vi "GoDef.vi"(8 "error in (no error)":errorcluster, 10 "String 2":string, 11 "QuickSilver in":refnum<class "QuickSilver.lvclass">) -> (0 "error out":errorcluster, 2 "String":string, 3 "QuickSilver out":refnum<class "QuickSilver.lvclass">)   [LabVIEW 2018, in "QuickSilver.lvclass"]
uses:
  QuickSilver.lvclass
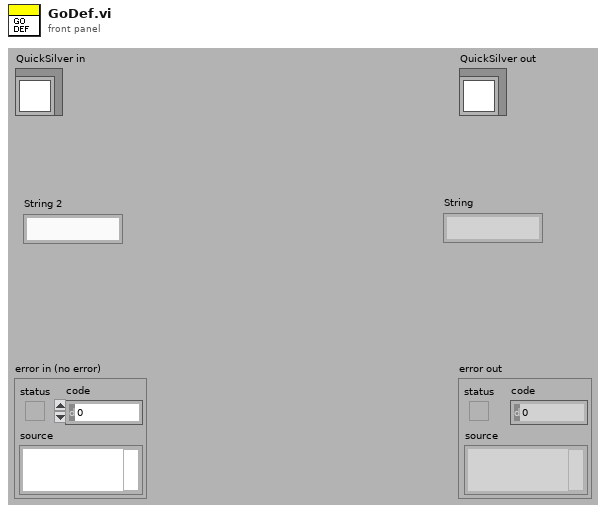
[diagram p1: front panel]
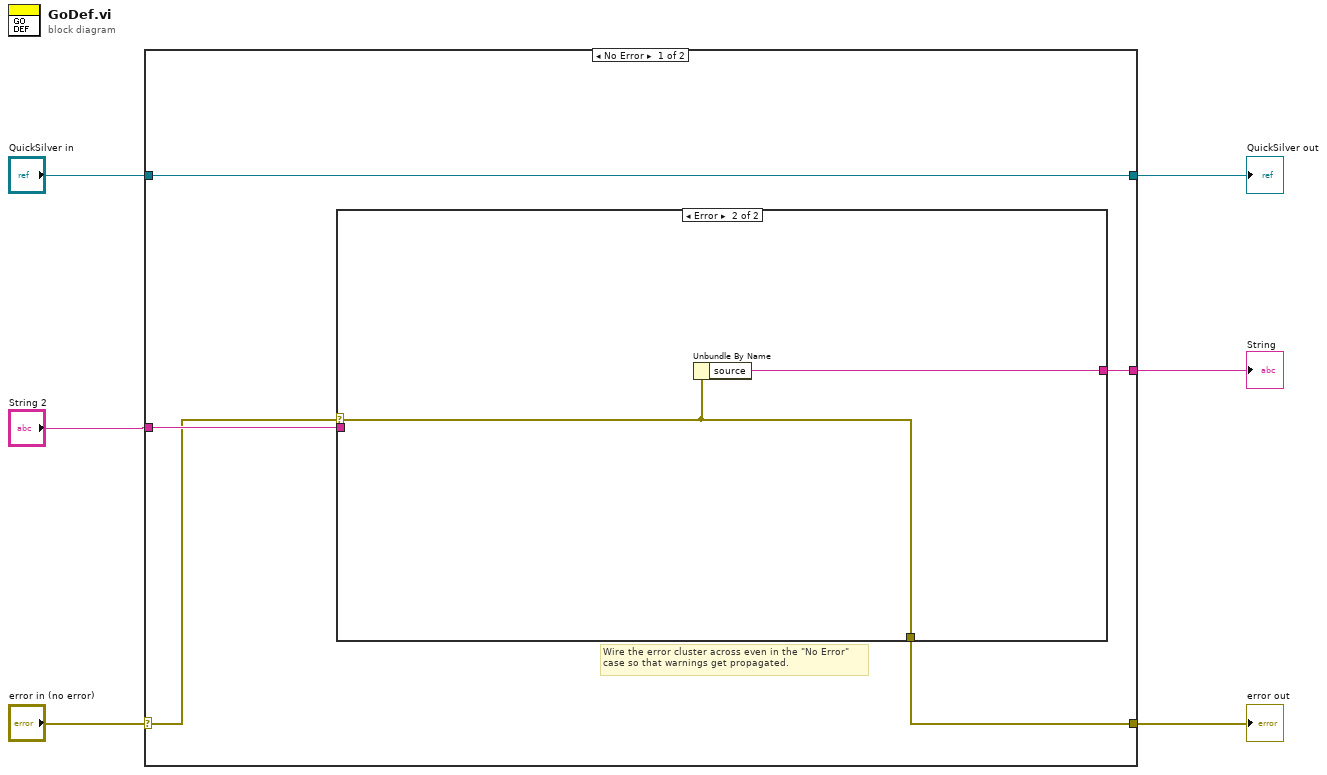
[diagram p0: block diagram]
diagram:
  n1 = case shown="No Error" "error in (no error)" {
    selector: "error in (no error)" -> [w7 w16]
    tunnel: [w9 w16] -> w1
    tunnel: [w8 w15] -> w3
    tunnel: "QuickSilver in" -> [w8 w15]
    tunnel: [w10 _] -> w2
    tunnel: "String 2" -> [w11 _]
    frame No Error {
      # "Wire the error cluster across even in the \"No Error\"\ncase so that warnings get propagated."
      n2 = case shown="Error" w7 {
        selector: w7 -> [w12 w13]
        tunnel: w11 -> [_ _]
        tunnel: [_ w14] -> w10
        tunnel: [w12 w13] -> w9
        frame No Error {
        }
        frame Error {
          n3 = Unbundle By Name(w13) -> ("source"=w14:string)
        }
      }
    }
    frame Error {
    }
  }
  "error out" <- w1
  "QuickSilver out" <- w3
  "String" <- w2
